vi "Actor Core.vi"(8 "error in":errorcluster, 11 "Nested in":refnum<class "BD_PAPAS_MEX_ESP.lvclass">) -> (0 "error out":errorcluster, 3 "Actor out":refnum<class "Actor.lvclass">)   [LabVIEW 2019, in "BD_PAPAS_MEX_ESP.lvlib" / "BD_PAPAS_MEX_ESP.lvclass"]
doc: "(<B>Filename</B>: Actor Framework.lvlib:Actor.lvclass:Actor Core.vi)\n\nReceives messages to the actor, reacts to them, and initiates any error handling that may shut the actor down.\n\nDescendant classes may override this VI to append parallel tasks for the actor to complete while it handles messages. Overrides use the Call Parent Method node."
uses:
  BD_PAPAS_MEX_ESP.lvclass
  C:/Program Files (x86)/National Instruments/LabVIEW 2019/vi.lib/ActorFramework/Actor/Actor.lvclass
  <vilib>/ActorFramework/Actor/Actor.lvclass
  BD_PAPAS_MEX_ESP.lvclass/BD_PAPAS_MEX_ESP.ctl
  <vilib>/ActorFramework/Actor/Actor.lvclass/Actor.ctl
  <vilib>/ActorFramework/Message Enqueuer/Message Enqueuer.lvclass/Message Enqueuer.ctl
  Write VI Refnum.vi
  <vilib>/ActorFramework/Message Enqueuer/Init from Existing Queue.vi
  <vilib>/ActorFramework/Message Enqueuer/Enqueue.vi
  <vilib>/ActorFramework/Stop Msg/Stop Msg.lvclass
  C:/Program Files (x86)/National Instruments/LabVIEW 2019/vi.lib/ActorFramework/Message/Message.lvclass
  <vilib>/ActorFramework/Message Priority Queue/Priority Enqueue.vi
  <vilib>/ActorFramework/Message Enqueuer/Message Enqueuer.lvclass
panel:
  in  "COMPRAR MERCANCÍA":bool
  in  "10 PESOS MEXICANOS":bool
  in  "5 PESOS MEXICANOS":bool
  in  "2 PESOS MEXICANOS":bool
  in  "1 PESO MEXICANO":bool
  out "CRÉDITO":dbl
  out "MONEDA":string
  out "PRODUCTO":string
  out "CANTIDAD":dbl
  out "PRECIO":dbl
  in  "SOLICITAR MERCANCIA":bool
  in  "MERCANCÍA":i32(listbox)
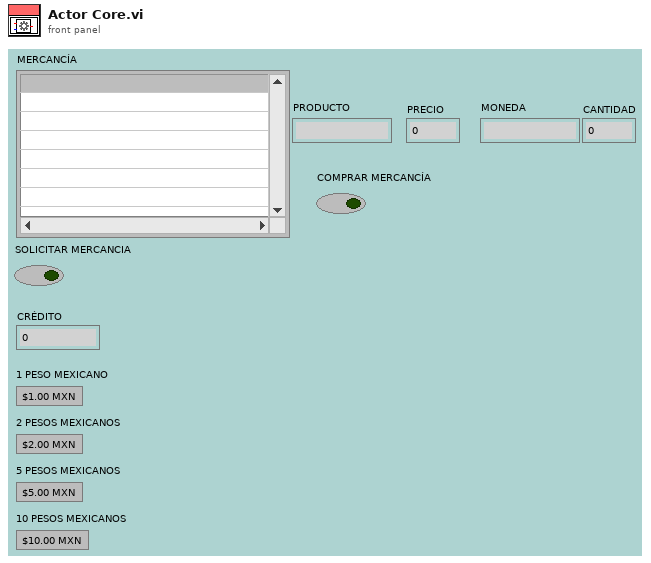
[diagram p1: front panel]
types:
  T1 = cluster{"CANTIDAD":dbl, "MONEDA":string, "PRECIO ":dbl, "PRODUCTO":string}
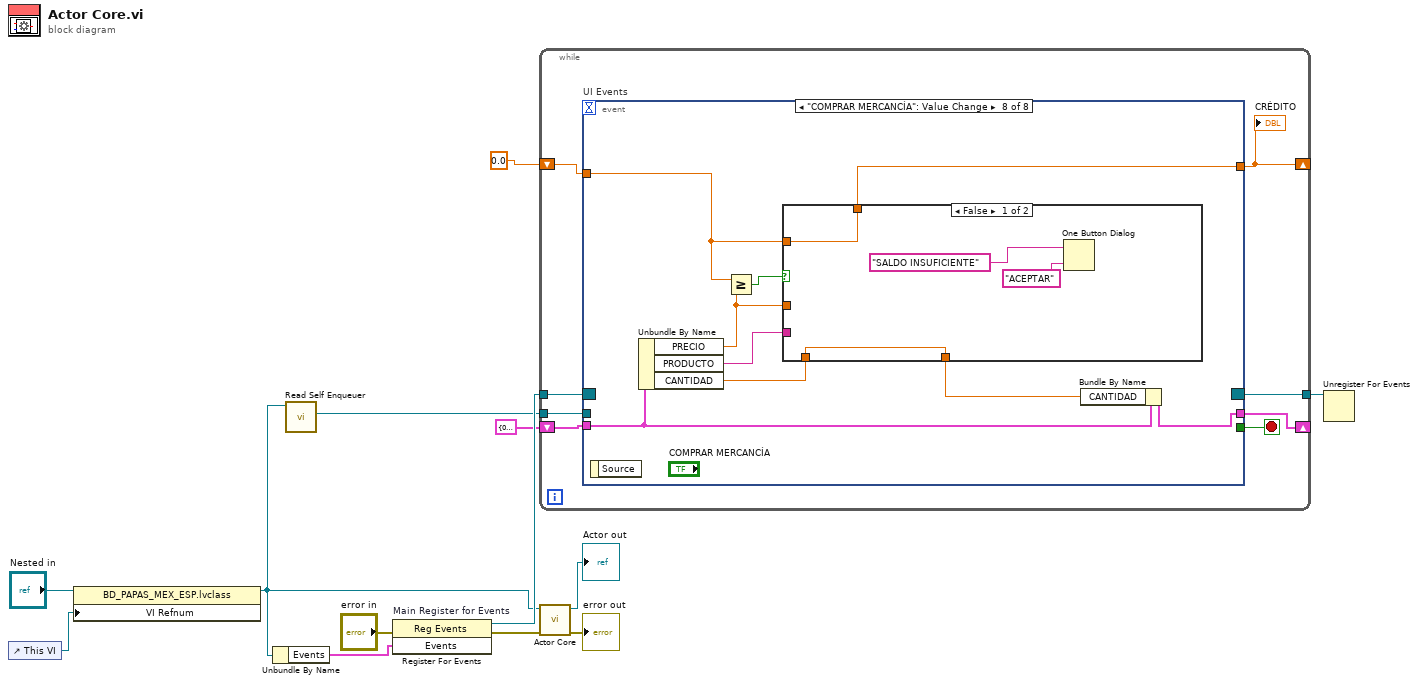
[diagram p0: block diagram]
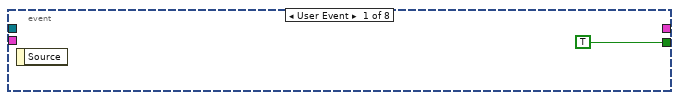
[diagram p2: hidden frame]
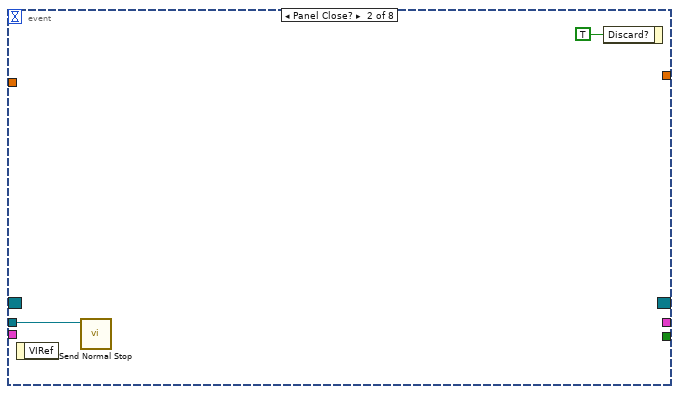
[diagram p3: hidden frame]
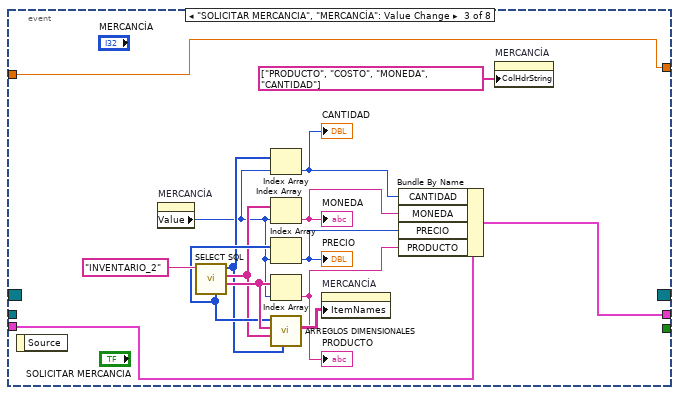
[diagram p4: hidden frame]
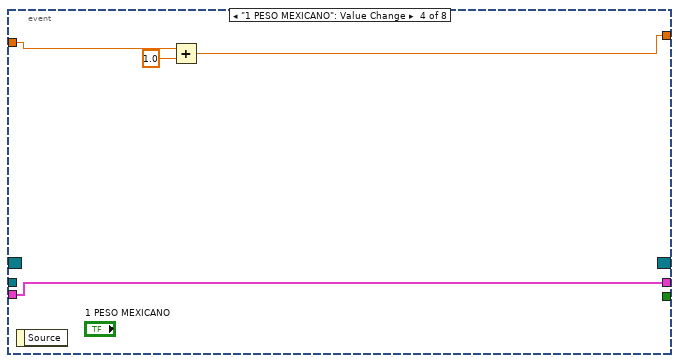
[diagram p5: hidden frame]
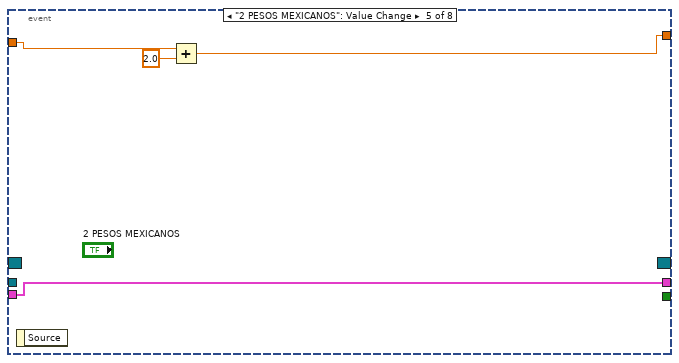
[diagram p6: hidden frame]
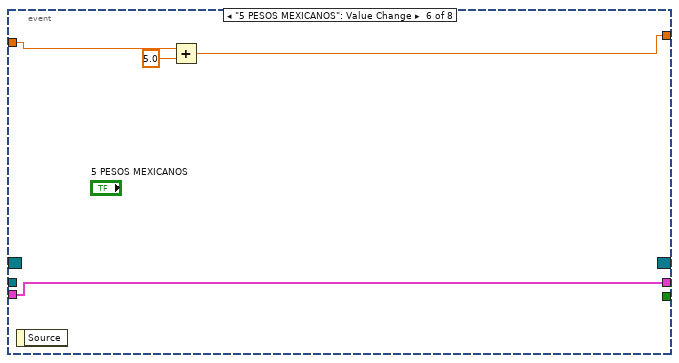
[diagram p7: hidden frame]
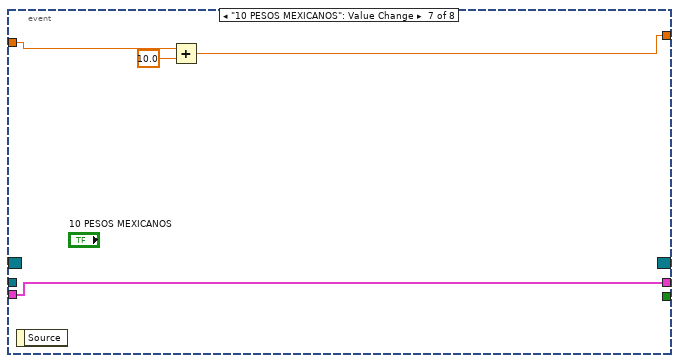
[diagram p8: hidden frame]
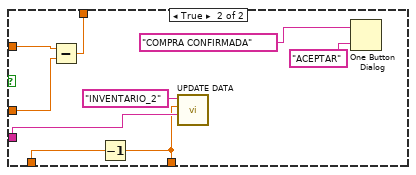
[diagram p9: hidden frame]
diagram:
  n1 = control-ref of="This VI"() -> (w3:refnum<vi>)
  n2 = property class="BD_PAPAS_MEX_ESP.lvclass"(reference="Nested in", "VI Refnum"=w3) -> (reference out=w4:refnum<class "BD_PAPAS_MEX_ESP.lvclass">)  [unwired: 1 in, 1 out]
  n3 = Unbundle By Name(w4) -> ("Events"=w10:cluster{"Stop":refnum<user-event>})
  n4 = call <vilib>:"Read Self Enqueuer.vi"("Actor"=w4) -> ("Self Enqueuer"=w7:refnum<class "Message Enqueuer.lvclass">)  [unwired: 10 in]
  n5 = register-events "Main Register for Events"(error in="error in", w10) -> (reference out=w11:refnum<event-registration>, error out=w5:errorcluster)  [unwired: 1 in]
  n6 = while {
    tunnel: w11 -> [w21]
    tunnel: [w19] -> w9
    tunnel: w7 -> [w18]
    shift-right: [w16] -> _
    shift-left: T1 {"CANTIDAD"=0.0, "MONEDA"="", "PRECIO "=0.0, "PRODUCTO"=""} -> [w17]
    shift-right: [w14] -> _
    shift-left: 0.0 ("CRÉDITO") -> [w15]
    stop <- w20 stop-if-true
    n7 = event "UI Events" shown="[7] \"COMPRAR MERCANCÍA\": Value Change" {
      selector: w21 -> [_ _ _ _ _ _ _ _]
      dyn-events: [_ _ _ _ _ _ _ _] -> w19
      timeout: _ -> [_ _ _ _ _ _ _ _]
      tunnel: [TRUE _ _ _ _ _ _ _] -> w20
      tunnel: w18 -> [_ w23 _ _ _ _ _ _]
      tunnel: w17 -> [_ _ w32 w43 w47 w51 w55 w64]
      tunnel: [_ _ w31 w43 w47 w51 w55 w60] -> w16
      tunnel: [_ _ w25 w40 w44 w48 w52 w56] -> w14
      tunnel: w15 -> [_ _ w25 w42 w46 w50 w54 w58]
      event User Event {
        n8 = event-data() -> ()  [unwired: 1 in, 1 out]
      }
      event Panel Close? {
        n9 = event-data() -> ()  [unwired: 1 in, 1 out]
        n10 = call <vilib>:"Send Normal Stop.vi"("Message Enqueuer"=w23) -> ()  [unwired: 10 in, 1 out]
        n11 = event-data("Discard?"=TRUE) -> ()  [unwired: 1 in, 1 out]
      }
      event "SOLICITAR MERCANCIA", "MERCANCÍA": Value Change {
        n12 = event-data() -> ()  [unwired: 1 in, 1 out]
        n13 = property on="MERCANCÍA" class="MCListbox (strict)"() -> ("Value"=w26:i32)  [unwired: 2 in, 2 out]
        n14 = call "SELECT SQL.vi"("INVENTARIO"="INVENTARIO_2") -> ("PRODUCTO"=w38:string[], "MONEDA"=w36:string[], "CANTIDAD"=w35:i64[], "COSTO"=w37:i64[])  [unwired: 7 in]
        n15 = Index Array(array=w35, index=w26) -> (element=w30:i64)
        "CANTIDAD" <- w30
        n16 = Index Array(array=w36, index=w26) -> (element=w29:string)
        "MONEDA" <- w29
        n17 = Index Array(array=w37, index=w26) -> (element=w28:i64)
        "PRECIO" <- w28
        n18 = Index Array(array=w38, index=w26) -> (element=w27:string)
        "PRODUCTO" <- w27
        n19 = call "ARREGLOS DIMENSIONALES.vi"("CANTIDAD"=w35, "MONEDA"=w36, "PRODUCTO"=w38, "COSTO"=w37) -> ("Array"=w33:string[][])  [unwired: 7 in]
        n20 = property on="MERCANCÍA" class="MCListbox (strict)"("ItemNames"=w33) -> ()  [unwired: 2 in, 2 out]
        n21 = Bundle By Name(cluster=w32, "CANTIDAD"=w30, "MONEDA"=w29, "PRECIO"=w28, "PRODUCTO"=w27) -> (w31:T1)
        n22 = property on="MERCANCÍA" class="MCListbox (strict)"("ColHdrString"=string[] ["PRODUCTO", "COSTO", "MONEDA", "CANTIDAD"] ("Column Header Strings[]")) -> ()  [unwired: 2 in, 2 out]
      }
      event "1 PESO MEXICANO": Value Change {
        n23 = event-data() -> ()  [unwired: 1 in, 1 out]
        n24 = Add(x=w42, y=1.0) -> (x+y=w40:dbl)
      }
      event "2 PESOS MEXICANOS": Value Change {
        n25 = event-data() -> ()  [unwired: 1 in, 1 out]
        n26 = Add(x=w46, y=2.0) -> (x+y=w44:dbl)
      }
      event "5 PESOS MEXICANOS": Value Change {
        n27 = event-data() -> ()  [unwired: 1 in, 1 out]
        n28 = Add(x=w50, y=5.0) -> (x+y=w48:dbl)
      }
      event "10 PESOS MEXICANOS": Value Change {
        n29 = event-data() -> ()  [unwired: 1 in, 1 out]
        n30 = Add(x=w54, y=10.0) -> (x+y=w52:dbl)
      }
      event "COMPRAR MERCANCÍA": Value Change {
        n31 = event-data() -> ()  [unwired: 1 in, 1 out]
        n32 = Unbundle By Name(w64) -> ("PRECIO"=w57:dbl, "PRODUCTO"=w61:string, "CANTIDAD"=w62:dbl)
        n33 = Greater Or Equal?(x=w58, y=w57) -> (x >= y?=w63:bool)
        n34 = case shown="False" w63 {
          tunnel: w62 -> [w67 w73]
          tunnel: w61 -> [_ w74]
          tunnel: [w67 w72] -> w59
          tunnel: w58 -> [w68 w71]
          tunnel: w57 -> [_ w70]
          tunnel: [w68 w69] -> w56
          frame False {
            n35 = One Button Dialog(message="SALDO INSUFICIENTE", button name ("OK")="ACEPTAR") -> ()  [unwired: 1 out]
          }
          frame True {
            n36 = Subtract(x=w71, y=w70) -> (x-y=w69:dbl)
            n37 = Decrement(x=w73) -> (x-1=w72:dbl)
            n38 = call "UPDATE DATA.vi"("PRODUCTO"=w74, "number"=w72, "TABLA"="INVENTARIO_2") -> ()  [unwired: 9 in]
            n39 = One Button Dialog(message="COMPRA CONFIRMADA", button name ("OK")="ACEPTAR") -> ()  [unwired: 1 out]
          }
        }
        n40 = Bundle By Name(cluster=w64, "CANTIDAD"=w59) -> (w60:T1)
      }
    }
    "CRÉDITO" <- w14
  }
  n41 = call-parent "Actor Core.vi"("error in"=w5, "Actor in"=w4) -> ("error out"=→"error out":errorcluster, "Actor out"=→"Actor out":refnum<class "Actor.lvclass">)  [unwired: 8 in]
  n42 = Unregister For Events(event registration refnum=w9) -> ()  [unwired: 1 in, 1 out]
